vi "http 414 Request URI Too Long.vi"(11 "application request in":T3) -> (3 "application request out":T1)   [LabVIEW 2013]
uses:
  http request.ctl
  http method.ctl
  http response.ctl
  http response packet type.ctl
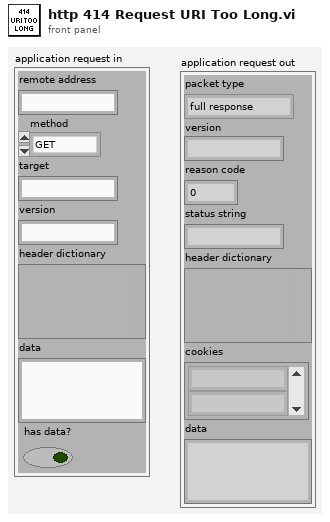
[diagram p1: front panel]
types:
  T1 = typedef "http response.ctl" = cluster{"packet type":T2, "version":string, "reason code":u16, "status string":string, "header dictionary":variant, "cookies":string[], "data":string}
  T2 = typedef "http response packet type.ctl" = enum16{"full response", "header only", "data only", "last data"}
  T3 = typedef "http request.ctl" = cluster{"remote address":string, "method":T4, "target":string, "version":string, "header dictionary":variant, "data":string, "has data?":bool}
  T4 = typedef "http method.ctl" = enum16{"GET", "POST", "PUT", "DELETE", "HEAD", "OPTIONS"}
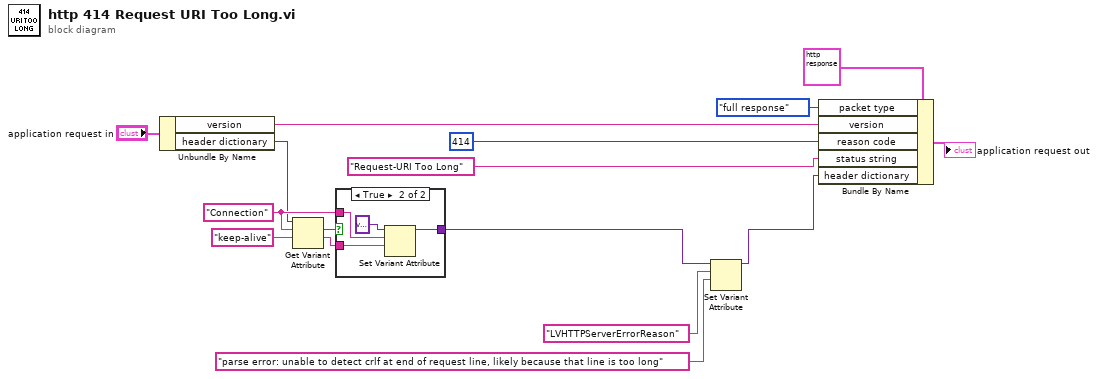
[diagram p0: block diagram]
diagram:
  w14 = "Connection" ("name")
  n1 = Unbundle By Name("application request in") -> ("version"=w10:string, "header dictionary"=w11:variant)
  n2 = Get Variant Attribute(Variant=w11, name=w14, default value (empty Variant)="keep-alive" ("name")) -> (found=w6:bool, value=w13:string)  [unwired: 1 in, 2 out]
  n3 = case shown="True" w6 {
    tunnel: [_ w20] -> w3
    tunnel: w14 -> [_ w19]
    tunnel: w13 -> [_ w18]
    frame False {
    }
    frame True {
      n4 = Set Variant Attribute(Variant=variant ("variant"), name=w19, value=w18) -> (Variant out=w20:variant)  [unwired: 1 in, 2 out]
    }
  }
  n5 = Set Variant Attribute(Variant=w3, name="LVHTTPServerErrorReason", value="parse error: unable to detect crlf at end of request line, likely because that line is too long" ("name")) -> (Variant out=w4:variant)  [unwired: 1 in, 2 out]
  n6 = Bundle By Name(cluster=T1 {"packet type"=enum."full response", "version"="", "reason code"=0, "status string"="", "header dictionary"=variant, "cookies"=[], "data"=""} ("application request"), "packet type"=http_response_packet_type."full response", "version"=w10, "reason code"=u16 414, "status string"="Request-URI Too Long", "header dictionary"=w4) -> (→"application request out":T1)
